vi "Handle Error -8996.vi"(8 "Tx Error":errorcluster, 10 "LNA Return Message Msg":refnum<class "LNA Return Message Msg.lvclass">, 11 "Message Enqueuer in":refnum<class "Message Enqueuer.lvclass">) -> (0 "Error Out":errorcluster)   [LabVIEW 2014, in "CS++LNA.lvlib"]
doc: "Send LNA Return Message Msg object with error info to message enqueuer (typically self enqueuer).\n\nHandle error code -8996 set in CS++LNAMessage.lvclass:Do.vi:\nMessage returned from RLNA, not found or bad typecast. (Sender)"
uses:
  CS++LNA.lvlib
  <vilib>/ActorFramework/Message Enqueuer/Message Enqueuer.lvclass
  <vilib>/NI/Actors/Linked Network Actor/Linked Network Actor Messages/LNA Return Message Msg/LNA Return Message Msg.lvclass
  <vilib>/NI/Actors/Linked Network Actor/Linked Network Actor Messages/LNA Return Message Msg/LNA Return Message Msg.lvclass/LNA Return Message Msg.ctl
  <vilib>/ActorFramework/Message Enqueuer/Message Enqueuer.lvclass/Message Enqueuer.ctl
  <vilib>/ActorFramework/Message Priority Queue/Priority Enqueue.vi
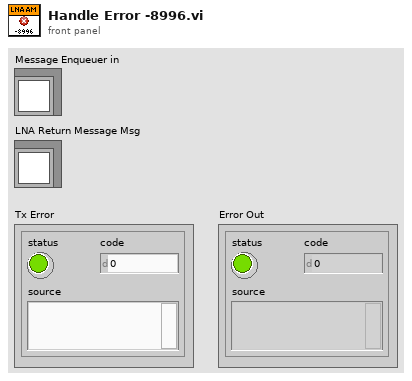
[diagram p1: front panel]
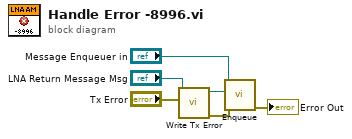
[diagram p0: block diagram]
diagram:
  n1 = call <vilib>:"Write Tx Error.vi"("Tx Error"="Tx Error", "LNA Return Message Msg in"="LNA Return Message Msg") -> ("error out"=w3:errorcluster, "LNA Return Message Msg out"=w6:refnum<class "LNA Return Message Msg.lvclass">)  [unwired: 8 in]
  n2 = call <vilib>:"Enqueue.vi"("error in (no error)"=w3, "Message"=w6, "Message Enqueuer in"="Message Enqueuer in") -> ("error out"=→"Error Out":errorcluster)  [unwired: 7 in, 1 out]
